vi "SParmSetup.vi"(0 "VISA IN":refnum<visa-resource-name>, 1 "Start Frequency":dbl=1000000000.0, 2 "Stop Frequency":dbl=2000000000.0, 3 "Filename":string="GainMag", 4 "Measurement":string(combo)="S22", 5 "Average?":bool=TRUE, 6 "AVG Factor":i32=20, 7 "error in":errorcluster, 8 "Autoscale?":bool=TRUE, 9 "Trace":i32=1, 10 "Points":dbl=201.0, 11 "Window":i32=1, 12 "IF BW":dbl, 13 "Channel":i32=1, 14 "Format":string(combo)="MLINear", 15 "Sweep Type":string(combo)="LINear", 17 "Power Level":dbl) -> (20 "VISA Out":refnum<visa-resource-name>, 27 "error out":errorcluster)   [LabVIEW 2018]
uses:
  PNA-X.lvlib
panel:
  in  "Ref Position":i32=5
  in  "Ref Level":i32=-10
  in  "Scale Per Division":i32=10
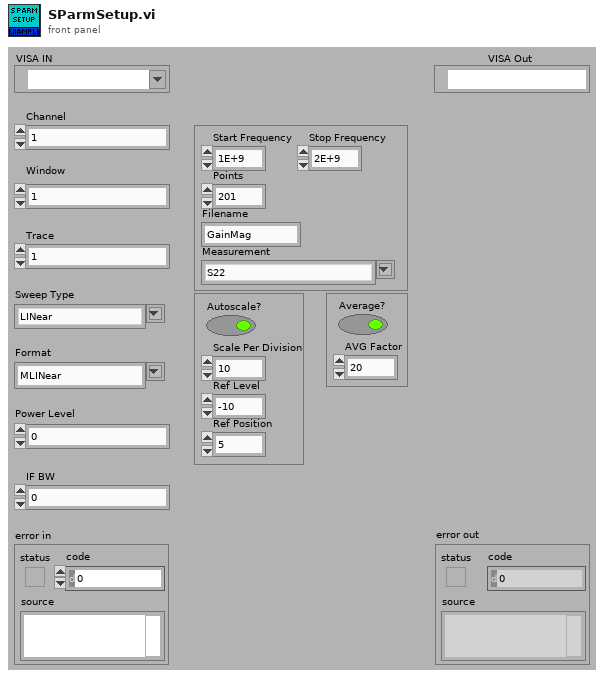
[diagram p1: front panel]
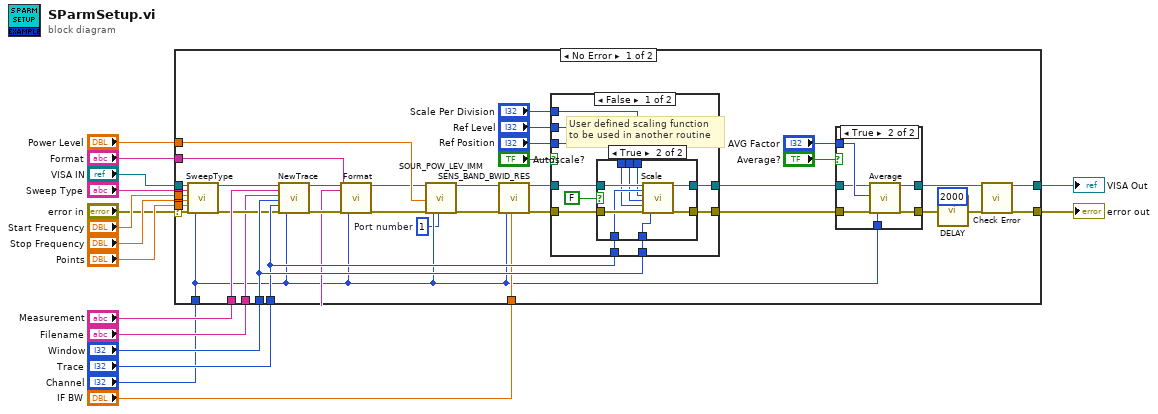
[diagram p0: block diagram]
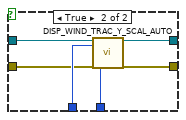
[diagram p4: hidden frame]
diagram:
  n1 = case shown="No Error" "error in" {
    selector: "error in" -> [w18 w92]
    tunnel: [w55 w91] -> w16
    tunnel: [w54 w92] -> w15
    tunnel: "Stop Frequency" -> [w53 _]
    tunnel: "Points" -> [w52 _]
    tunnel: "Sweep Type" -> [w51 _]
    tunnel: "Start Frequency" -> [w50 _]
    tunnel: "Measurement" -> [w49 _]
    tunnel: "Window" -> [w48 _]
    tunnel: "Trace" -> [w47 _]
    tunnel: "VISA IN" -> [w35 w91]
    tunnel: "Power Level" -> [w33 _]
    tunnel: "IF BW" -> [w28 _]
    tunnel: "Filename" -> [w21 _]
    tunnel: "Channel" -> [w20 _]
    tunnel: "Format" -> [w19 _]
    frame No Error {
      w17 = 1  # Port number
      n2 = call "SweepType.vi"("VISA IN"=w35, "Sweep Type"=w51, "Start Frq."=w50, "Stop Frq."=w53, "Points"=w52, "error in"=w18, "Channel"=w20) -> ("VISA Out"=w23:refnum<visa-resource-name>, "error out"=w22:errorcluster)  [unwired: 11 in]
      n3 = call "NewTrace.vi"("VISA IN"=w23, "Measurement"=w49, "FileName"=w21, "Window"=w48, "Trace"=w47, "error in (no error)"=w22, "Channel"=w20) -> ("VISA Out"=w26:refnum<visa-resource-name>, "error out"=w27:errorcluster)  [unwired: 11 in]
      n4 = call "Format.vi"("VISA IN"=w26, "Measurement Name"=w21, "Format"=w19, "error in"=w27, "Channel"=w20) -> ("VISA Out"=w24:refnum<visa-resource-name>, "error out"=w25:errorcluster)  [unwired: 13 in]
      n5 = call "SOUR_POW_LEV_IMM.vi"("VISA IN"=w24, "Power Level"=w33, "error in"=w25, "Channel"=w20, "Port number"=w17) -> ("VISA Out"=w31:refnum<visa-resource-name>, "error out"=w32:errorcluster)  [unwired: 13 in]
      n6 = call "SENS_BAND_BWID_RES.vi"("VISA IN"=w31, "error in"=w32, "Channel"=w20, "Resolution"=w28) -> ("VISA Out"=w30:refnum<visa-resource-name>, "error out"=w29:errorcluster)  [unwired: 14 in]
      n7 = case shown="False" "Autoscale?" {
        tunnel: w29 -> [w72 w87]
        tunnel: w30 -> [w73 w88]
        tunnel: w47 -> [w69 w89]
        tunnel: w48 -> [w68 w90]
        tunnel: [w70 w85] -> w45
        tunnel: [w71 w86] -> w34
        tunnel: "Scale Per Division" -> [w67 _]
        tunnel: "Ref Level" -> [w66 _]
        tunnel: "Ref Position" -> [w65 _]
        frame False {
          # "User defined scaling function\nto be used in another routine"
          n8 = case shown="True" FALSE {
            tunnel: w73 -> [w75 w84]
            tunnel: w72 -> [w74 w83]
            tunnel: [w74 w82] -> w71
            tunnel: [w75 w81] -> w70
            tunnel: w69 -> [_ w80]
            tunnel: w68 -> [_ w79]
            tunnel: w67 -> [_ w78]
            tunnel: w66 -> [_ w77]
            tunnel: w65 -> [_ w76]
            frame False {
            }
            frame True {
              n9 = call "Scale.vi"("VISA IN"=w84, "Trace"=w80, "Scale Per Division"=w78, "Ref Level"=w77, "Ref Position"=w76, "error in"=w83, "Window"=w79) -> ("VISA Out"=w81:refnum<visa-resource-name>, "error out"=w82:errorcluster)  [unwired: 11 in]
            }
          }
        }
        frame True {
          n10 = call "DISP_WIND_TRAC_Y_SCAL_AUTO.vi"("VISA IN"=w88, "Trace"=w89, "error in"=w87, "Window"=w90) -> ("VISA Out"=w85:refnum<visa-resource-name>, "error out"=w86:errorcluster)  [unwired: 14 in]
        }
      }
      n11 = case shown="True" "Average?" {
        tunnel: w45 -> [w57 w58]
        tunnel: w34 -> [w56 w63]
        tunnel: [w56 w62] -> w41
        tunnel: [w57 w61] -> w42
        tunnel: w20 -> [_ w60]
        tunnel: "AVG Factor" -> [_ w59]
        frame False {
        }
        frame True {
          n12 = call "Average.vi"("VISA IN"=w58, "AVG"=w59, "error in"=w63, "Channel"=w60) -> ("VISA Out"=w61:refnum<visa-resource-name>, "error out"=w62:errorcluster)  [unwired: 14 in]
        }
      }
      n13 = call "DELAY.vi"("milliseconds to wait"=u32 2000, "error in (no error)"=w41) -> ("error out"=w40:errorcluster)  [unwired: 13 in]
      n14 = call "Check Error.vi"("VISA Resource Name"=w42, "error in (no error)"=w40) -> ("dup VISA session"=w55:refnum<visa-resource-name>, "error out"=w54:errorcluster)  [unwired: 16 in]
    }
    frame Error {
    }
  }
  "VISA Out" <- w16
  "error out" <- w15
